vi "DAQFileIO.vi"(6 "Aquire Data":bool, 8 "error in (no error)":errorcluster, 9 "File Path In":path, 10 "Names":string[](array[string])=["Resistance (Ohms)", "Ethanol (%)", "RH (%)", "Temp (C)", "MFC A", "MFC B"], 11 "data":waveform(dbl)[](array[waveform])) -> (0 "error out":errorcluster, 1 "file path out":path)   [LabVIEW 2020]
panel:
  in  "Names":string[](array[string])=["Resistance (Ohms)", "Ethanol (%)", "RH (%)", "Temp (C)", "MFC A", "MFC B"]
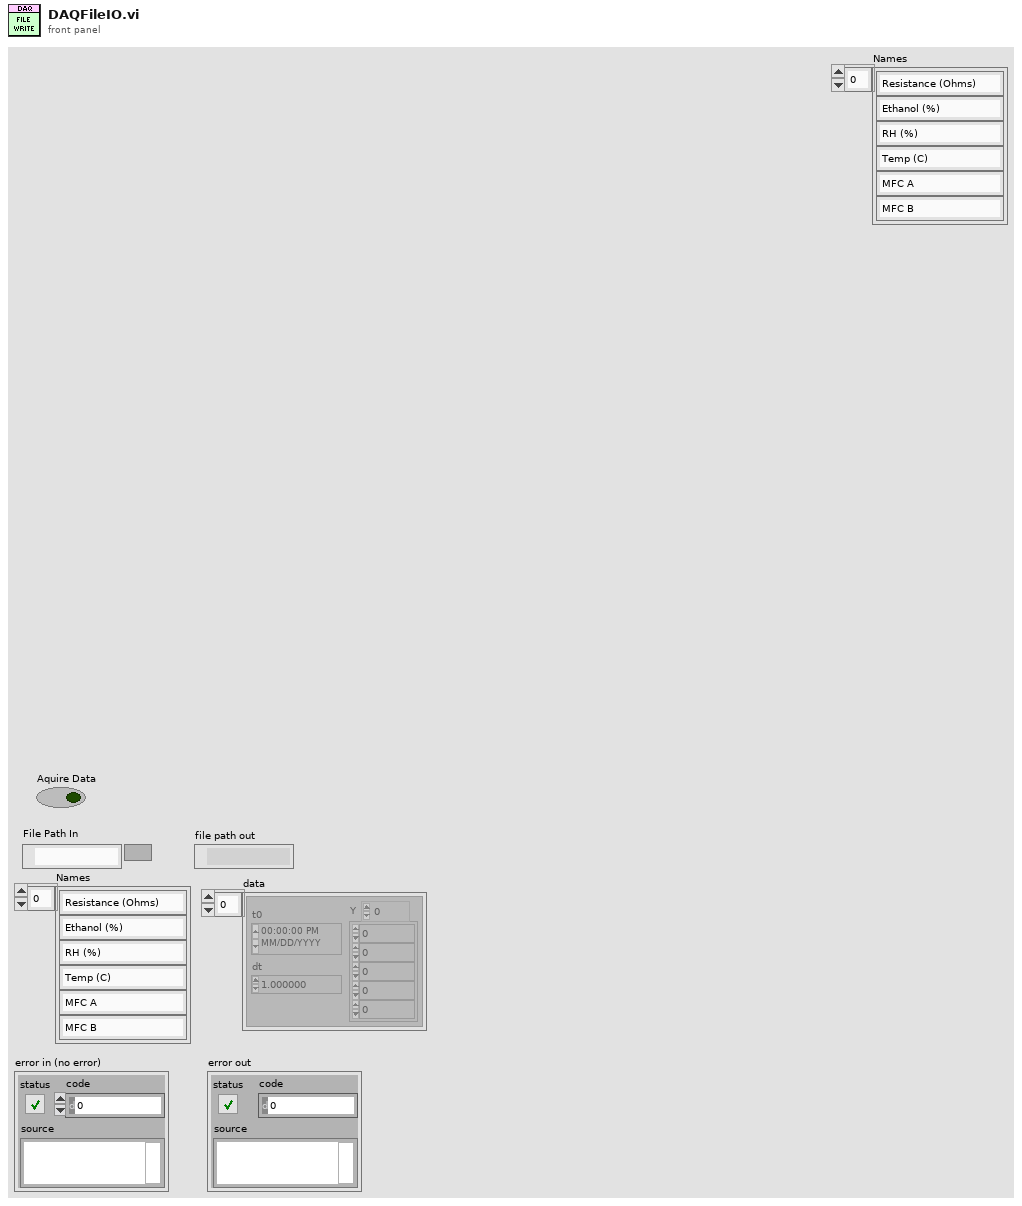
[diagram p1: front panel]
types:
  T1 = enum16{"open", "open or create", "create or replace", "create", "open (read-only)"}
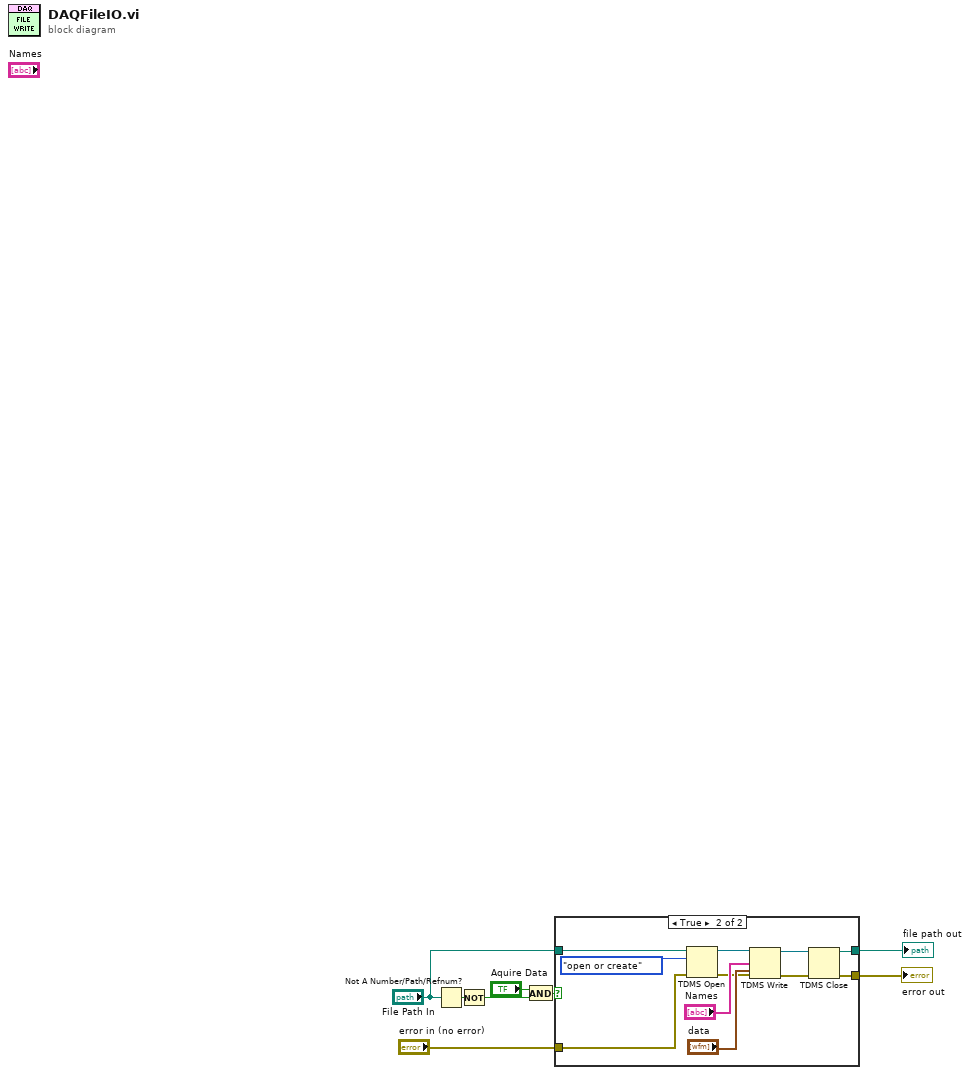
[diagram p0: block diagram]
diagram:
  n1 = Not A Number/Path/Refnum?(number/path/refnum="File Path In") -> (NaN/Path/Refnum?=w5:bool)
  n2 = Not(x=w5) -> (.not. x?=w6:bool)
  n3 = And(x="Aquire Data", y=w6) -> (x .and. y?=w8:bool)
  n4 = case shown="True" w8 {
    tunnel: [w10 w14] -> w3
    tunnel: "File Path In" -> [w10 w21]
    tunnel: [w9 w13] -> w2
    tunnel: "error in (no error)" -> [w9 w12]
    frame False {
    }
    frame True {
      n5 = TDMS Open(8:w12, 10:T1."open or create" ("operation (0:open)"), 11:w21) -> (0:w17:errorcluster, 3:w20:refnum<k34>)  [unwired: 4 in]
      n6 = TDMS Write(0:w20, 7:"Names", 9:"data", 11:w17) -> (4:w15:refnum<k34>, 15:w16:errorcluster)  [unwired: 2 in, 2 out]
      n7 = TDMS Close(8:w16, 11:w15) -> (0:w13:errorcluster, 3:w14:path)
    }
  }
  "file path out" <- w3
  "error out" <- w2
